vi "PC_Test_Network_Variables.vi"() -> ()   [LabVIEW 2020]
uses:
  <vilib>/dex/Stream Element Allocation Mode.ctl
  <vilib>/Waveform/WDTOps.llb/WDT Get Final Time Value DBL.vi
panel:
  in  "stop":bool
  out "Waveform Chart 2":waveform(dbl)(graph)
  out "Waveform Chart":waveform(i32)(graph)
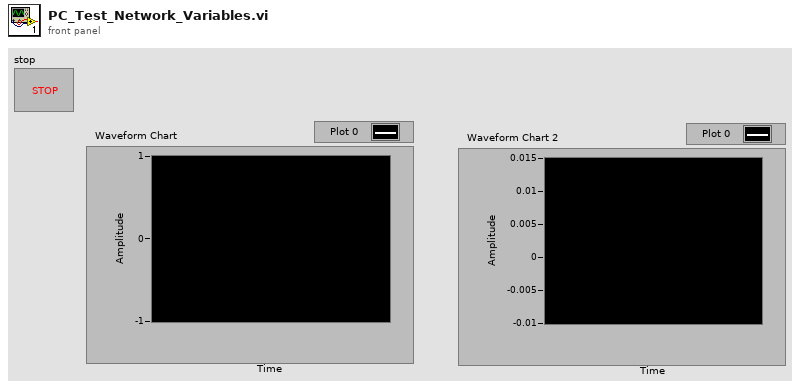
[diagram p1: front panel]
types:
  T1 = typedef "Stream Element Allocation Mode.ctl" = u32
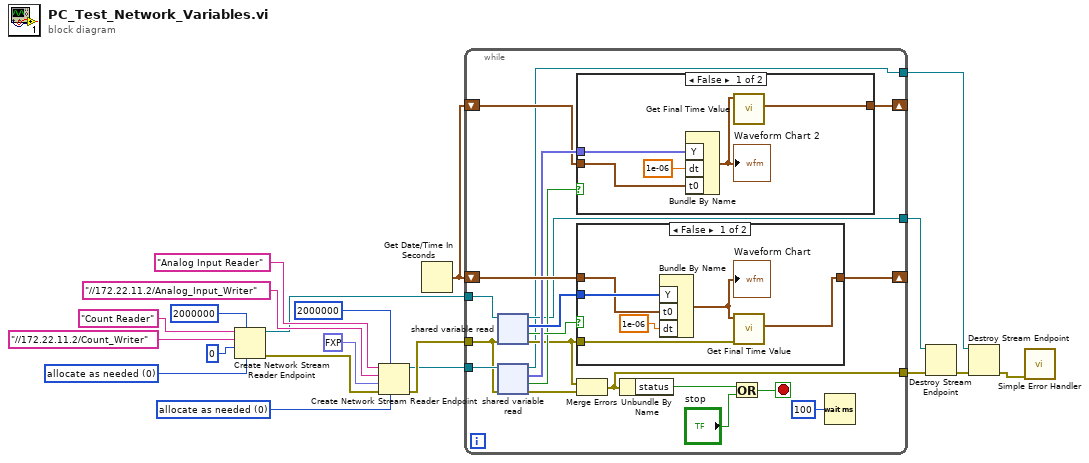
[diagram p0: block diagram]
diagram:
  w14 = T1 0 items=["allocate as needed", "pre-allocate"] ("element allocation mode")
  w17 = T1 0 items=["allocate as needed", "pre-allocate"] ("element allocation mode")
  n1 = Create Network Stream Reader Endpoint(6:w17, 7:2000000 ("reader buffer size"), 9:0, 10:"//172.22.11.2/Count_Writer" ("writer url"), 11:"Count Reader" ("reader name")) -> (0:w11:errorcluster, 3:w10:refnum<k21>)  [unwired: 2 in]
  n2 = Create Network Stream Reader Endpoint(6:w14, 7:2000000 ("reader buffer size"), 8:w11, 9:fxp<+/-,17,5> 0.0, 10:"//172.22.11.2/Analog_Input_Writer" ("writer url"), 11:"Analog Input Reader" ("reader name")) -> (0:w9:errorcluster, 3:w8:refnum<k21>)  [unwired: 1 in]
  n3 = Get Date/Time In Seconds() -> (seconds since 1Jan1904=w6:timestamp)
  n4 = while {
    shift-right: [w37] -> _
    shift-left: w6 -> [w38]
    tunnel: w10 -> [w40]
    tunnel: w9 -> [w35]
    tunnel: w8 -> [w36]
    shift-right: [w32] -> _
    shift-left: w6 -> [w33]
    tunnel: [w24] -> w4
    tunnel: [w23] -> w5
    tunnel: [w22] -> w3
    stop <- w25 stop-if-true
    n5 = shared-variable-read(w40, w35) -> (w23:refnum<k21>, w29:errorcluster, w31:bool, w39:i32[])  [unwired: 2 in]
    n6 = shared-variable-read(w36, w35) -> (w22:refnum<k21>, w28:errorcluster, w30:bool, w34:fxp<+/-,17,5>[])  [unwired: 2 in]
    n7 = case shown="False" w30 {
      tunnel: w34 -> [w45 _]
      tunnel: w33 -> [w43 w46]
      tunnel: [w42 w46] -> w32
      frame False {
        n8 = Bundle By Name("Y"=w45, "dt"=1e-06, "t0"=w43) -> (w41:waveform(dbl))  [unwired: 1 in]
        "Waveform Chart 2" <- w41
        n9 = call-poly <vilib>:"Get Final Time Value.vi"("waveform in"=w41) -> ("tf"=w42:timestamp)  [unwired: 8 in, 2 out]
      }
      frame True {
      }
    }
    n10 = case shown="False" w31 {
      tunnel: w39 -> [w52 _]
      tunnel: w38 -> [w51 w53]
      tunnel: [w48 w53] -> w37
      tunnel: w29 -> [w47 _]
      frame False {
        n11 = Bundle By Name("Y"=w52, "t0"=w51, "dt"=1e-06) -> (w49:waveform(i32))  [unwired: 1 in]
        "Waveform Chart" <- w49
        n12 = call-poly <vilib>:"Get Final Time Value.vi"("error in (no error)"=w47, "waveform in"=w49) -> ("tf"=w48:timestamp)  [unwired: 7 in, 2 out]
      }
      frame True {
      }
    }
    n13 = Merge Errors(w29, w28) -> (w24:errorcluster)
    n14 = Unbundle By Name(w24) -> ("status"=w26:bool)
    n15 = Or(x=w26, y="stop") -> (x .or. y?=w25:bool)
    n16 = Wait (ms)(milliseconds to wait=u32 100) -> ()  [unwired: 1 out]
  }
  n17 = Destroy Stream Endpoint(8:w4, 11:w5) -> (0:w2:errorcluster)
  n18 = Destroy Stream Endpoint(8:w2, 11:w3) -> (0:w1:errorcluster)
  n19 = call <vilib>:"Simple Error Handler.vi"("error in (no error)"=w1) -> ()  [unwired: 4 in, 5 out]
